vi "2039_hw INAVUpdatePosition.vi"() -> ()   [LabVIEW 2016, in "2039lib.lvlib"]
uses:
  2039lib.lvlib
  <vilib>/Rock Robotics/WPI/Gyro/WPI_GyroDevRef.ctl
  <vilib>/Rock Robotics/SystemInterfaces/AI/FPGA_AIChannel.ctl
  <vilib>/Rock Robotics/SystemInterfaces/spilib/spi_bus.ctl
  <vilib>/Rock Robotics/WPI/Accelerometer/WPI_AccelerometerDevRef.ctl
  <vilib>/Rock Robotics/WPI/Accelerometer/WPI_AccelerometerScaling.ctl
  <vilib>/Rock Robotics/WPI/Accelerometer/WPI_AccelerometerAnalogChannels.ctl
  <vilib>/Rock Robotics/SystemInterfaces/i2clib/i2c_bus.ctl
  <vilib>/Rock Robotics/WPI/Accelerometer/ADXL345 Range.ctl
  <vilib>/Rock Robotics/WPI/Accelerometer/WPI_AccelerometerADXL345 Axes.ctl
panel:
  in  "Rightward Direction":T1(ring)
  in  "Forward Direction":enum16{"X Forward", "Y Forward", "Z Forward"}(ring)
  in  "INAV Sensor Cluster":T11 {"GyroDevRef"."Sample Rate" min=0.25 max=100.0 step=0.25; "AccelerometerDevRef"."Device Address" format="%.0x"; "AccelerometerDevRef"."Accel Range" items=["+/- 2 g", "+/- 4 g", "+/- 8 g", "+/- 16 g"]}
  # "Analog"
  # "XRS"
  # "ADXL"
  # "Analog"
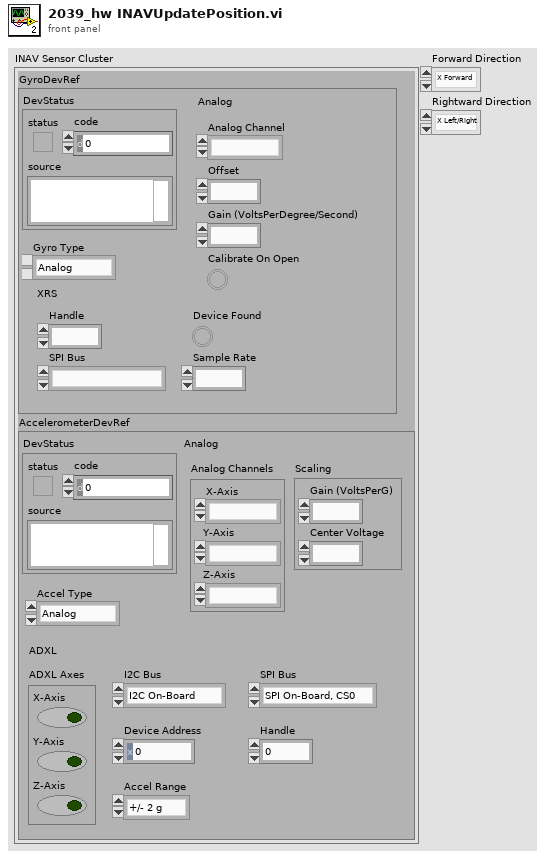
[diagram p1: front panel]
types:
  T1 = enum16{"X Left/Right", "Y Left/Right", "Z Left/Right"}
  T2 = typedef "WPI_GyroDevRef.ctl" = cluster{"DevStatus":errorcluster, "Analog Channel":T3, "Offset":dbl, "Gain (VoltsPerDegree/Second)":dbl, "Gyro Type":enum16{"Analog", "XRS450"}, "Handle":i32, "SPI Bus":T4, "Device Found":bool, "Sample Rate":dbl, "Calibrate On Open":bool}
  T3 = typedef "FPGA_AIChannel.ctl" = enum8{"AI 0", "AI 1", "AI 2", "AI 3", "AI MXP 0", "AI MXP 1", "AI MXP 2", "AI MXP 3", "Invalid"}
  T4 = typedef "spi_bus.ctl" = enum16{"SPI On-Board, CS0", "SPI On-Board, CS1", "SPI On-Board, CS2", "SPI On-Board, CS3", "SPI MXP", "Invalid"}
  T5 = typedef "WPI_AccelerometerDevRef.ctl" = cluster{"DevStatus":errorcluster, "Scaling":T6, "Analog Channels":T7, "I2C Bus":T8, "SPI Bus":T4, "Accel Range":T9, "ADXL Axes":T10, "Handle":i32, "Device Address":u8, "Accel Type":enum16{"Analog", "ADXL345 I2C", "ADXL345 SPI", "Internal", "ADXL362 SPI"}}
  T6 = typedef "WPI_AccelerometerScaling.ctl" = cluster{"Gain (VoltsPerG)":dbl, "Center Voltage":dbl}
  T7 = typedef "WPI_AccelerometerAnalogChannels.ctl" = cluster{"X-Axis":T3, "Y-Axis":T3, "Z-Axis":T3}
  T8 = typedef "i2c_bus.ctl" = enum16{"I2C On-Board", "I2C MXP", "Invalid"}
  T9 = typedef "ADXL345 Range.ctl" = u8
  T10 = typedef "WPI_AccelerometerADXL345 Axes.ctl" = cluster{"X-Axis":bool, "Y-Axis":bool, "Z-Axis":bool}
  T11 = cluster{"GyroDevRef":T2, "AccelerometerDevRef":T5}
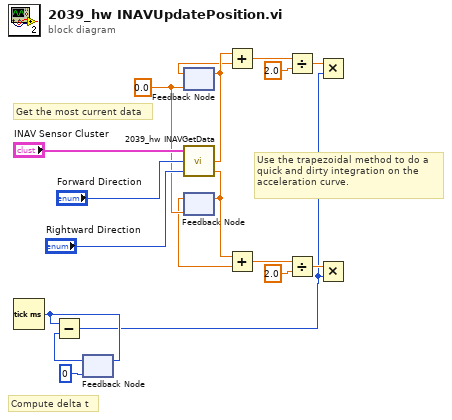
[diagram p0: block diagram]
diagram:
  w15 = 0.0
  # "Use the trapezoidal method to do a\nquick and dirty integration on the \nacceleration curve."
  # "Compute delta t"
  # "Get the most current data"
  n1 = Tick Count (ms)() -> (millisecond timer value=w3:u32)
  n2 = feedback #1(u32 0 ("millisecond timer value")) -> (w2:u32)
  n3 = Subtract(x=w3, y=w2) -> (x-y=w1:u32)
  n4 = feedback-in #1(w3) -> ()
  n5 = feedback #2(w15) -> (w13:dbl)
  n6 = call "2039_hw INAVGetData.vi"("Rightward Direction"="Rightward Direction", "Forward Direction"="Forward Direction", "INAV Sensor Cluster"="INAV Sensor Cluster") -> ("Rightward Accel"=w12:dbl, "Forward Accel"=w14:dbl)  [unwired: 1 out]
  n7 = feedback-in #2(w14) -> ()
  n8 = feedback-in #3(w12) -> ()
  n9 = feedback #3(w15) -> (w11:dbl)
  n10 = Add(x=w14, y=w13) -> (x+y=w10:dbl)
  n11 = Add(x=w12, y=w11) -> (x+y=w9:dbl)
  n12 = Divide(x=w10, y=2.0) -> (x/y=w6:dbl)
  n13 = Divide(x=w9, y=2.0) -> (x/y=w5:dbl)
  n14 = Multiply(x=w6, y=w1) -> ()  [unwired: 1 out]
  n15 = Multiply(x=w5, y=w1) -> ()  [unwired: 1 out]
